vi "Vision Processing - Test.vi"(8 "error in (no error)":errorcluster, 11 "Image Size":T1=enum."320x240") -> ()   [LabVIEW 2016]
uses:
  Vision Support Code/Camera Types.ctl
  <vilib>/Rock Robotics/WPI/Camera/WPI_CameraImageSize.ctl
  <vilib>/Rock Robotics/WPI/Camera/WPI_CameraWhite Balance Values.ctl
  <vilib>/Rock Robotics/WPI/Camera/WPI_CameraExposure Values.ctl
  <vilib>/Rock Robotics/WPI/Camera/WPI_CameraFrameRate.ctl
  TestBuild/Robot Global Data - Test.vi
  <vilib>/Rock Robotics/Network Tables/NT Write Number.vi
  <vilib>/vision/NI_Vision_Development_Module.lvlib
panel:
  in  "Image Size 2":T1=enum."320x240"
  out "loop ms":u32=74
  out "Calibration error":errorcluster={"status"=TRUE, "code"=-1074396113, "source"=""}
  in  "Display Original":bool
  in  "Display Mask":bool=TRUE
  in  "Line Border":cluster{"Top":dbl, "Bottom":dbl}={"Top"=6.0, "Bottom"=1.0}
  in  "Use Calibration":bool=TRUE
  out "Instructions:":string="Use Source to load image files from a directory, or use a USB or IP camera connected to your laptop. Use Camera Settings 1 and 2 to achieve a dark image with bright and colorful stripes.\nLED Color can encoded as HSL or related color modes. Calibrate to the same color as the strips being reflected to the camera.\nClick and draw a line in Original Image to auto-calibrate the LED Color. You may want to widen and tweak Sat and Val by hand.\nThe Annotate button affects drawing a rectangle around the stripes and labeling it with a distance in ft. Distance relies on knowing the Camera Type and lens calibration (it looks up the lens view angle).\n\nAdjust Score Cutoff to make the code more or less picky. If the color is not very unique, you may need to increase the number of particles considered. The diagram uses a Size Limit to ignore colored things that are too small. You may need to adjust it if you are targetting from far away.\n\nResults give you the distance to the target, the center and box in a normalized (-1 to 1) and pixel coordinates.\n\nBe sure to read about setting camera exposure and brightness to help simplify your image and acquire color saturated images.\n\nThere are lots of comments on the diagram to explain the code."
  in  "Color Mode":u16(ring)=3 items=["RGB", "HSL", "HSV", "HSI"]
  in  "Particles":dbl=5.0
  in  "Score Cutoff %":dbl=70.0
  in  "Camera Type":T2=enum."MS HD3000 square"
  out "Results":T3={"Distance (ft)"=inf, "Score"=-inf, "Normalized"={"Center"={-0.565625, 0.37083333333333335}, "Rectangle"={"Numeric"=-inf, "Numeric 2"=inf, "Numeric 3"=-inf, "Numeric 5"=inf}}, "Pixels"={"Center"={69.5, 75.5}, "Rectangle"={"Numeric"=-inf, "Numeric 2"=-inf, "Numeric 3"=-inf, "Numeric 5"=-inf}}} {"Score" format="%#_3g"; "Pixels"."Rectangle"."Numeric 5" format="%#_3g"; "Pixels"."Rectangle"."Numeric 3" format="%#_3g"; "Pixels"."Rectangle"."Numeric 2" format="%#_3g"; "Pixels"."Rectangle"."Numeric" format="%#_3g"; "Normalized"."Rectangle"."Numeric 5" format="%#_2g"; "Normalized"."Rectangle"."Numeric 3" format="%#_2g"; "Normalized"."Rectangle"."Numeric 2" format="%#_2g"; "Normalized"."Rectangle"."Numeric" format="%#_2g"; "Normalized"."Center"."?" format="%#_3g"; "Normalized"."Center"."?" format="%#_3g"; "Distance (ft)" format="%#_3g"}
  out "Qualified Particles":i32=1
  in  "LED Color":T4={"Hue"={46.852959751357716, 116.77171286119035}, "Sat"={0.0, 255.0}, "Val"={15.178571428571438, 255.0}} {"Hue" scale=0.0..255.0 scale format="%#_3g"}
  out "Mask":T5(plugin-control)
  out "Original Image":T5(plugin-control)
  # "Legend:\n    Rectangle\n       Green - Good target, distance ft\n       Red - Bad target\n    Orange Text - Score in %"
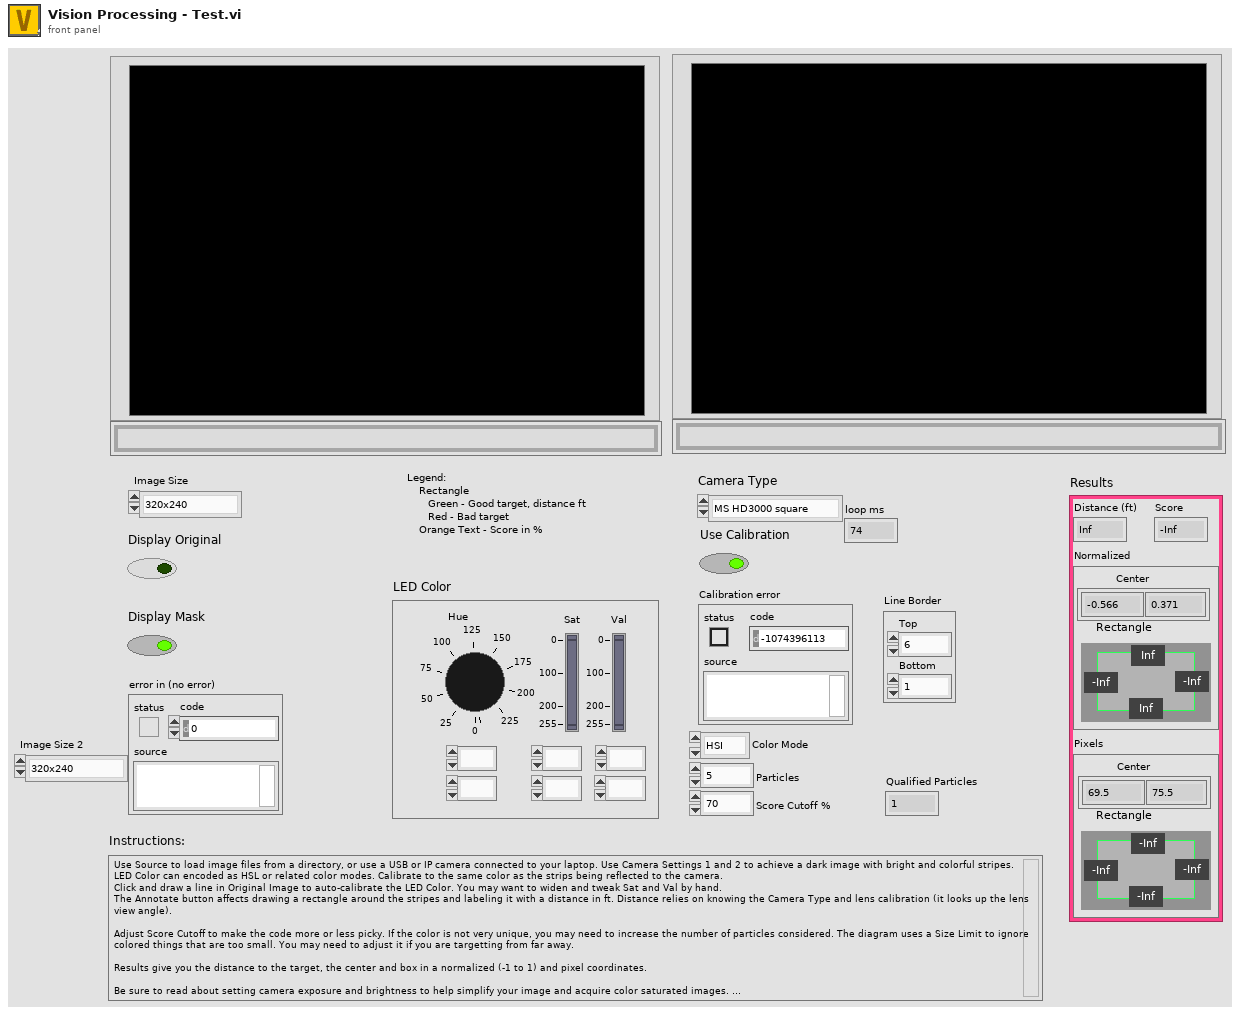
[diagram p1: front panel]
types:
  T1 = typedef "WPI_CameraImageSize.ctl" = enum16{"640x480", "320x240", "160x120", "Custom"}
  T2 = typedef "Camera Types.ctl" = enum16{"206", "1011", "1013", "MS HD3000 square", "MS HD3000 640x480"}
  T3 = cluster{"Distance (ft)":dbl, "Score":dbl, "Normalized":cluster{"Center":cluster{dbl, dbl}, "Rectangle":cluster{"Numeric":dbl, "Numeric 2":dbl, "Numeric 3":dbl, "Numeric 5":dbl}}, "Pixels":cluster{"Center":cluster{dbl, dbl}, "Rectangle":cluster{"Numeric":dbl, "Numeric 2":dbl, "Numeric 3":dbl, "Numeric 5":dbl}}}
  T4 = cluster{"Hue":cluster{dbl, dbl}, "Sat":cluster{dbl, dbl}, "Val":cluster{dbl, dbl}}
  T5 = typedef "IMAQ Image.ctl" = refnum<image>
  T6 = typedef "WPI_CameraFrameRate.ctl" = u32
  T7 = typedef "WPI_CameraExposure Values.ctl" = enum16{"Auto", "Flicker-free 50 Hz", "Flicker-free 60 Hz", "Hold current", "Custom"}
  T8 = typedef "WPI_CameraWhite Balance Values.ctl" = enum16{"Auto", "Fixed indoor", "Fixed outdoor 1", "Fixed outdoor 2", "Fixed fluorescent 1", "Fixed fluorescent 2", "Hold current", "Custom"}
  T9 = typedef "Image Type" = u32
  T10 = typedef "Particle Parameters" = i32
  T11 = typedef "WPI_CameraDevRef.ctl" = cluster{"Camera Address":string, "CameraStatus":errorcluster}
  T12 = cluster{"Left":dbl, "Top":dbl, "Right":dbl, "Bottom":dbl}
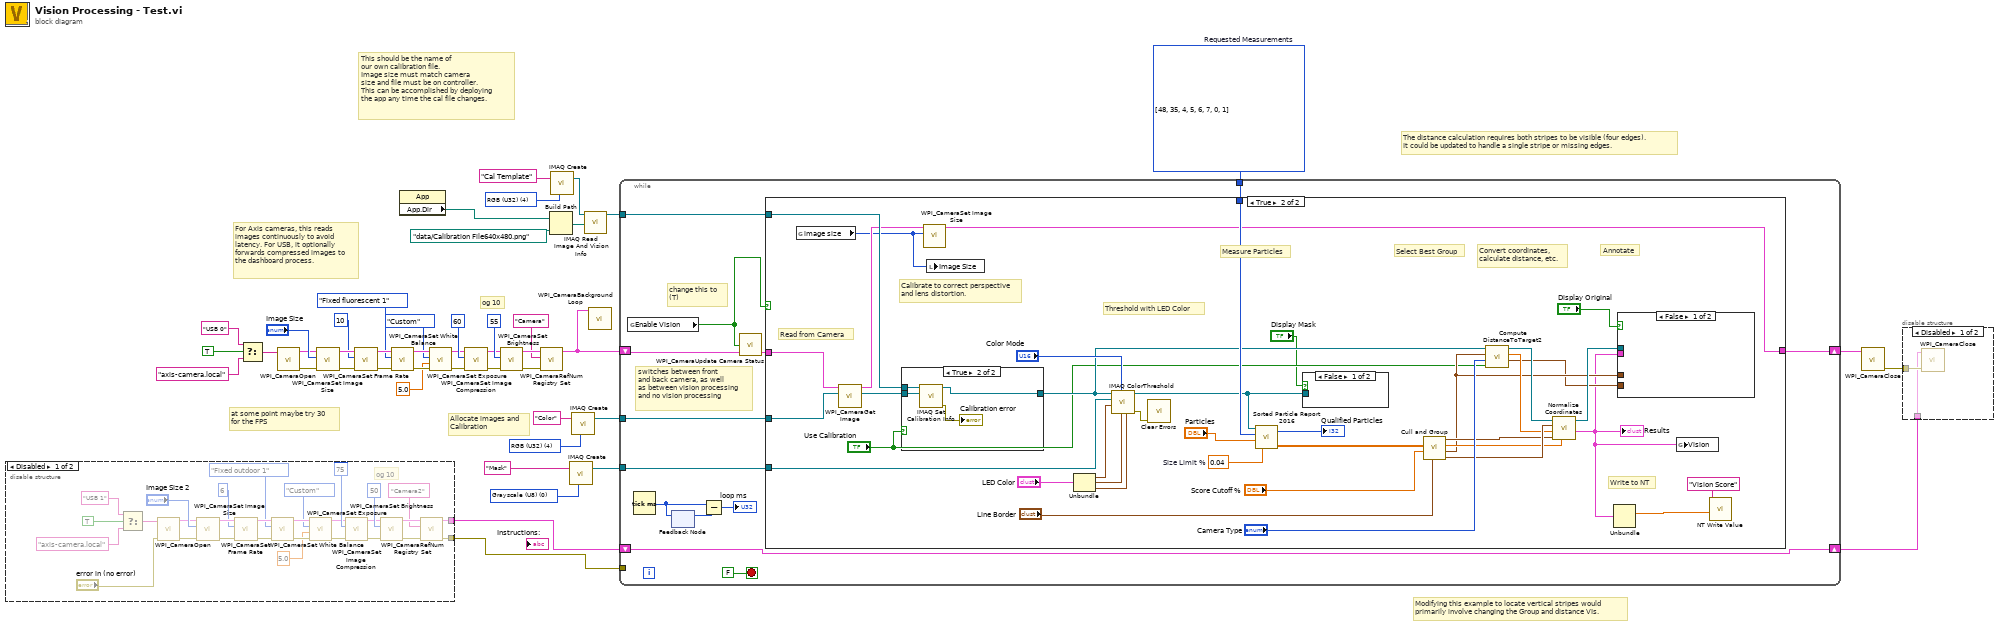
[diagram p0: block diagram]
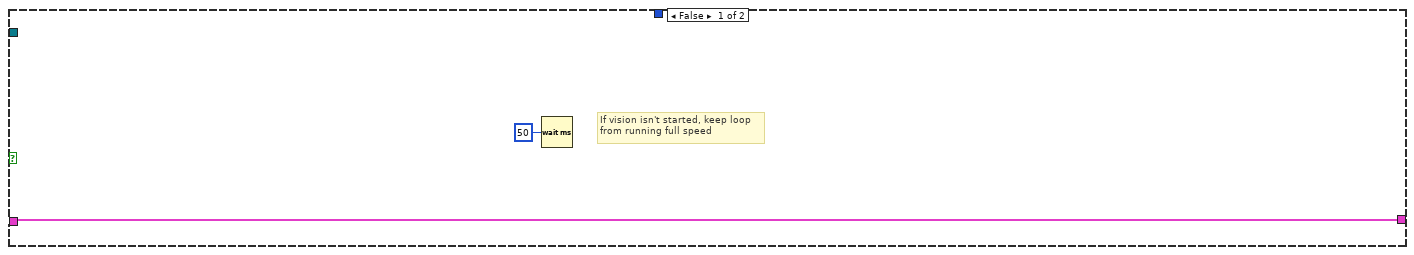
[diagram p4: hidden frame]
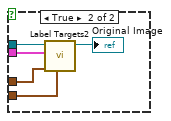
[diagram p5: hidden frame]
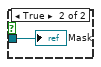
[diagram p6: hidden frame]
diagram:
  w39 = T9 4 items=["Grayscale (U8)", "Grayscale (I16)", "Grayscale (SGL)", "Complex (CSG)", "RGB (U32)", "HSL (U32)", "RGB (U64)", "Grayscale (U16)"] ("Image Type")
  w41 = T10[] [48, 35, 4, 5, 6, 7, 0, 1] items=["Center of Mass X", "Center of Mass Y", "First Pixel X", "First Pixel Y", "Bounding Rect Left", "Bounding Rect Top", "Bounding Rect Right", "Bounding Rect Bottom", "Max Feret Diameter Start X", "Max Feret Diameter Start Y", "Max Feret Diameter End X", "Max Feret Diameter End Y", "Max Horiz. Segment Length Left", "Max Horiz. Segment Length Right", "Max Horiz. Segment Length Row", "-", "Bounding Rect Width", "Bounding Rect Height", "Bounding Rect Diagonal", "Perimeter", "Convex Hull Perimeter", "Holes' Perimeter", "Max Feret Diameter", "Equivalent Ellipse Major Axis", "Equivalent Ellipse Minor Axis", "Equivalent Ellipse Minor Axis (Feret)", "Equivalent Rect Long Side", "Equivalent Rect Short Side", "Equivalent Rect Diagonal", "Equivalent Rect Short Side (Feret)", "Average Horiz. Segment Length", "Average Vert. Segment Length", "Hydraulic Radius", "Waddel Disk Diameter", "-", "Area", "Holes' Area", "Particle & Holes' Area", "Convex Hull Area", "Image Area", "-", "Number of Holes", "Number of Horiz. Segments", "Number of Vert. Segments", "-", "Orientation", "Max Feret Diameter Orientation", "-", "% Area/Image Area", "% Area/(Particle & Holes' Area)", "Ratio of Equivalent Ellipse Axes", "Ratio of Equivalent Rect Sides", "-", "Elongation Factor", "Compactness Factor", "Heywood Circularity Factor", "Type Factor", "-", "Sum X", "Sum Y", "Sum XX", "Sum XY", "Sum YY", "Sum XXX", "Sum XXY", "Sum XYY", "Sum YYY", "-", "Moment of Inertia XX", "Moment of Inertia XY", "Moment of Inertia YY", "Moment of Inertia XXX", "Moment of Inertia XXY", "Moment of Inertia XYY", "Moment of Inertia YYY", "Norm. Moment of Inertia XX", "Norm. Moment of Inertia XY", "Norm. Moment of Inertia YY", "Norm. Moment of Inertia XXX", "Norm. Moment of Inertia XXY", "Norm. Moment of Inertia XYY", "Norm. Moment of Inertia YYY", "Hu Moment 1", "Hu Moment 2", "Hu Moment 3", "Hu Moment 4", "Hu Moment 5", "Hu Moment 6", "Hu Moment 7"]  # Requested Measurements
  w44 = T9 0 items=["Grayscale (U8)", "Grayscale (I16)", "Grayscale (SGL)", "Complex (CSG)", "RGB (U32)", "HSL (U32)", "RGB (U64)", "Grayscale (U16)"] ("Image Type")
  w45 = T9 4 items=["Grayscale (U8)", "Grayscale (I16)", "Grayscale (SGL)", "Complex (CSG)", "RGB (U32)", "HSL (U32)", "RGB (U64)", "Grayscale (U16)"] ("Image Type")
  # "og 10"
  # "at some point maybe try 30 \nfor the FPS"
  # "This should be the name of \nour own calibration file.\nImage size must match camera\nsize and file must be on controller.\nThis can be accomplished by deploying\nthe app any time the cal file changes."
  # "For Axis cameras, this reads\nimages continuously to avoid\nlatency. For USB, it optionally\nforwards compressed images to\nthe dashboard process."
  # "Modifying this example to locate vertical stripes would\nprimarily involve changing the Group and distance VIs."
  # "The distance calculation requires both stripes to be visible (four edges).\nIt could be updated to handle a single stripe or missing edges."
  # "Allocate images and\nCalibration"
  n1 = disable-structure shown="Disabled" {
    disable-tunnel: [w49 _] -> w4
    disable-tunnel: [w47 _] -> w2
    frame Disabled {
      # "og 10"
      n2 = Select(t="USB 1" ("format string"), s=TRUE ("dot notation? (F)"), f="axis-camera.local" ("format string")) -> (s? t:f=w51:string)
      n3 = call <vilib>:"WPI_CameraOpen.vi"("error in (no error)"="error in (no error)", "Camera Address"=w51) -> ("error out"=w63:errorcluster, "CameraDevRef"=w64:T11)  [unwired: 8 out]
      n4 = call <vilib>:"WPI_CameraSet Image Size.vi"("error in (no error)"=w63, "Image Size"="Image Size 2", "CameraDevRef"=w64) -> ("error out"=w62:errorcluster, "CameraDevRef Out"=w65:T11)  [unwired: 1 in, 6 out]
      n5 = call <vilib>:"WPI_CameraSet Frame Rate.vi"("error in (no error)"=w62, "Frame Rate (fps)"=T6 6, "CameraDevRef"=w65) -> ("error out"=w61:errorcluster, "CameraDevRef Out"=w67:T11)  [unwired: 7 out]
      n6 = call <vilib>:"WPI_CameraSet White Balance.vi"("error in (no error)"=w61, "White Balance"=WPI_CameraWhite_Balance_Values."Fixed outdoor 1", "CameraDevRef"=w67) -> ("error out"=w60:errorcluster, "CameraDevRef Out"=w66:T11)  [unwired: 1 in, 6 out]
      n7 = call <vilib>:"WPI_CameraSet Exposure.vi"("error in (no error)"=w60, "Exposure (%)"=5.0, "Exposure"=WPI_CameraExposure_Values."Custom", "CameraDevRef"=w66) -> ("error out"=w59:errorcluster, "CameraDevRef Out"=w69:T11)  [unwired: 6 out]
      n8 = call <vilib>:"WPI_CameraSet Image Compression.vi"("error in (no error)"=w59, "Compression"=75, "CameraDevRef"=w69) -> ("error out"=w58:errorcluster, "CameraDevRef Out"=w68:T11)  [unwired: 7 out]
      n9 = call <vilib>:"WPI_CameraSet Brightness.vi"("error in (no error)"=w58, "Brightness"=50, "CameraDevRef"=w68) -> ("error out"=w57:errorcluster, "CameraDevRef Out"=w75:T11)  [unwired: 7 out]
      n10 = call <vilib>:"WPI_CameraRefNum Registry Set.vi"("error in (no error)"=w57, "refnum name"="Camera2", "CameraDevRef"=w75) -> ("error out"=w49:errorcluster, "CameraDevRef"=w47:T11)  [unwired: 1 in, 6 out]
    }
    frame Enabled {
    }
  }
  n11 = Select(t="USB 0" ("format string"), s=TRUE ("dot notation? (F)"), f="axis-camera.local" ("format string")) -> (s? t:f=w9:string)
  n12 = call <vilib>:"WPI_CameraOpen.vi"("Camera Address"=w9) -> ("error out"=w21:errorcluster, "CameraDevRef"=w22:T11)  [unwired: 1 in, 8 out]
  n13 = call <vilib>:"WPI_CameraSet Image Size.vi"("error in (no error)"=w21, "Image Size"="Image Size", "CameraDevRef"=w22) -> ("error out"=w20:errorcluster, "CameraDevRef Out"=w23:T11)  [unwired: 1 in, 6 out]
  n14 = call <vilib>:"WPI_CameraSet Frame Rate.vi"("error in (no error)"=w20, "Frame Rate (fps)"=T6 10, "CameraDevRef"=w23) -> ("error out"=w19:errorcluster, "CameraDevRef Out"=w25:T11)  [unwired: 7 out]
  n15 = call <vilib>:"WPI_CameraSet White Balance.vi"("error in (no error)"=w19, "White Balance"=WPI_CameraWhite_Balance_Values."Fixed fluorescent 1", "CameraDevRef"=w25) -> ("error out"=w18:errorcluster, "CameraDevRef Out"=w24:T11)  [unwired: 1 in, 6 out]
  n16 = property class="App"() -> ("App.Dir"=w5:path)  [unwired: 2 in, 2 out]
  n17 = call <vilib>:"WPI_CameraSet Exposure.vi"("error in (no error)"=w18, "Exposure (%)"=5.0, "Exposure"=WPI_CameraExposure_Values."Custom", "CameraDevRef"=w24) -> ("error out"=w17:errorcluster, "CameraDevRef Out"=w27:T11)  [unwired: 6 out]
  n18 = call <vilib>:"WPI_CameraSet Image Compression.vi"("error in (no error)"=w17, "Compression"=60, "CameraDevRef"=w27) -> ("error out"=w16:errorcluster, "CameraDevRef Out"=w26:T11)  [unwired: 7 out]
  n19 = call <vilib>:"WPI_CameraSet Brightness.vi"("error in (no error)"=w16, "Brightness"=55, "CameraDevRef"=w26) -> ("error out"=w15:errorcluster, "CameraDevRef Out"=w33:T11)  [unwired: 7 out]
  n20 = call <vilib>:"WPI_CameraRefNum Registry Set.vi"("error in (no error)"=w15, "refnum name"="Camera", "CameraDevRef"=w33) -> ("CameraDevRef"=w8:T11)  [unwired: 1 in, 7 out]
  n21 = Build Path(base path=w5, name or relative path=path "data/Calibration File640x480.png" ("Folder Location")) -> (appended path=w35:path)
  n22 = call "IMAQ Create"("Image Name"="Cal Template", "Image Type"=w39) -> ("New Image"=w37:T5)  [unwired: 2 in, 2 out]
  n23 = call "IMAQ Create"("Image Name"="Mask", "Image Type"=w44) -> ("New Image"=w42:T5)  [unwired: 2 in, 2 out]
  n24 = call "IMAQ Create"("Image Name"="Color", "Image Type"=w45) -> ("New Image"=w40:T5)  [unwired: 2 in, 2 out]
  n25 = call "IMAQ Read Image And Vision Info"("File Path"=w35, "Image"=w37) -> ("Image Out"=w36:T5)  [unwired: 7 in, 2 out]
  n26 = call <vilib>:"WPI_CameraBackground Loop.vi"("CameraDevRef"=w8) -> ()  [unwired: 11 in]
  n27 = while {
    tunnel: w40 -> [w84]
    tunnel: w42 -> [w87]
    tunnel: w41 -> [w86]
    tunnel: w36 -> [w85]
    shift-right: [w83] -> w7
    shift-left: w8 -> [w82]
    tunnel: w4 -> [_]
    shift-right: [w76] -> w1
    shift-left: w2 -> [w76]
    stop <- FALSE stop-if-true
    # "change this to \n(T)"
    # "switches between front\nand back camera, as well \nas between vision processing \nand no vision processing"
    n28 = global read "Robot Global Data - Test.vi" "Enable Vision"() -> (w77:bool)
    n29 = Tick Count (ms)() -> (millisecond timer value=w79:u32)
    n30 = feedback-in #1(w79) -> ()
    n31 = feedback #1() -> (w80:u32)  [unwired: 1 in]
    n32 = Subtract(x=w79, y=w80) -> (x-y=→"loop ms":u32)
    n33 = call <vilib>:"WPI_CameraUpdate Camera Status.vi"("CameraDevRef In"=w82, "Enable Vision"=w77) -> ("CameraDevRef Out"=w81:T11)  [unwired: 3 in]
    n34 = case shown="True" w77 {
      tunnel: w87 -> [_ w128]
      tunnel: w86 -> [_ w124]
      tunnel: w85 -> [_ w104]
      tunnel: w81 -> [w90 w101]
      tunnel: w84 -> [_ w100]
      tunnel: [w90 w95] -> w83
      frame False {
        # "If vision isn't started, keep loop\nfrom running full speed"
        n35 = Wait (ms)(milliseconds to wait=u32 50) -> ()  [unwired: 1 out]
      }
      frame True {
        w122 = 0.04  # Size Limit %
        # "Write to NT"
        # "Read from Camera"
        # "Calibrate to correct perspective\nand lens distortion."
        # "Measure Particles"
        # "Convert coordinates,\ncalculate distance, etc."
        # "Annotate"
        # "Select Best Group"
        # "Threshold with LED Color"
        n36 = global read "Robot Global Data - Test.vi" "image size"() -> (w94:T1)
        n37 = call <vilib>:"WPI_CameraGet Image.vi"("Image"=w100, "CameraDevRef"=w101) -> ("Image Out"=w99:T5, "CameraDevRef Out"=w96:T11)  [unwired: 7 in, 1 out]
        n38 = case shown="True" "Use Calibration" {
          tunnel: [w135 w139] -> w105
          tunnel: w99 -> [w135 w138]
          tunnel: w104 -> [_ w137]
          frame False {
          }
          frame True {
            n39 = call "IMAQ Set Calibration Info"("Image Dst"=w138, "Image Src"=w137) -> ("error out"=→"Calibration error":errorcluster, "Calibrated Image"=w139:T5)  [unwired: 8 in]
          }
        }
        n40 = call <vilib>:"WPI_CameraSet Image Size.vi"("Image Size"=w94, "CameraDevRef"=w96) -> ("CameraDevRef Out"=w95:T11)  [unwired: 2 in, 7 out]
        n41 = local write "Image Size"(w94) -> ()
        n42 = Unbundle("LED Color") -> ("Hue"=w127:cluster{dbl, dbl}, "Sat"=w126:cluster{dbl, dbl}, "Val"=w125:cluster{dbl, dbl})
        n43 = call "IMAQ ColorThreshold"("Blue or Luma or Val or Inten Range"=w125, "Green or Sat Range"=w126, "Color Mode"="Color Mode", "Red or Hue Range"=w127, "Image Dst"=w128, "Image Src"=w105) -> ("error out"=w121:errorcluster, "Image Dst Out"=w117:T5)  [unwired: 4 in]
        n44 = call <vilib>:"Clear Errors.vi"("error in (no error)"=w121) -> ()  [unwired: 5 in, 2 out]
        n45 = call "Sorted Particle Report 2016.vi"("Min Area Size %"=w122, "Particle Count Limit"="Particles", "Pixel Measurements"=w124, "Image in"=w117) -> ("Sorted Data"=w119:dbl[][], "Particles"=→"Qualified Particles":i32)
        n46 = case shown="False" "Display Mask" {
          tunnel: w117 -> [_ w134]
          frame False {
          }
          frame True {
            "Mask" <- w134
          }
        }
        n47 = call "Cull and Group.vi"("Line Border"="Line Border", "Score Cutoff"="Score Cutoff %", "Sorted Data"=w119) -> ("Rect"=w115:T12, "Line"=w107:T12, "Score"=w110:dbl, "Center"=w111:cluster{"X":dbl, "Y":dbl})  [unwired: 5 in]
        n48 = call "Compute DistanceToTarget2.vi"("Calibrated"="Use Calibration", "Camera Type"="Camera Type", "Line"=w107, "Image Src"=w105) -> ("Edges"=w106:cluster{"X":sgl, "Y":sgl}[], "Distance (ft)"=w114:dbl, "Image Dst Out"=w113:T5)  [unwired: 5 in]
        n49 = call "Normalize Coordinates.vi"("Score"=w110, "Center"=w111, "Distance"=w114, "Bounding box"=w115, "Image in"=w113) -> ("Results"=w91:T3, "Image out"=w112:T5)  [unwired: 5 in]
        "Results" <- w91
        n50 = Unbundle(w91) -> ("Score"=w93:dbl)  [unwired: 3 out]
        n51 = case shown="False" "Display Original" {
          tunnel: w112 -> [_ w132]
          tunnel: w91 -> [_ w131]
          tunnel: w107 -> [_ w130]
          tunnel: w106 -> [_ w129]
          frame False {
          }
          frame True {
            n52 = call "Label Targets2.vi"("Edges"=w129, "Line"=w130, "Results"=w131, "Image in"=w132) -> ("Image out"=→"Original Image":T5)  [unwired: 7 in]
          }
        }
        n53 = global write "Robot Global Data - Test.vi" "Vision"(w91) -> ()
        n54 = call-poly <vilib>:"NT Write Value.vi"("Numeric"=w93, "Name"="Vision Score") -> ()  [unwired: 9 in, 1 out]
      }
    }
  }
  n55 = call <vilib>:"WPI_CameraClose.vi"("CameraDevRef"=w7) -> ("error out"=w3:errorcluster)  [unwired: 1 in, 9 out]
  n56 = disable-structure shown="Disabled" {
    disable-tunnel: w3 -> [w141 _]
    disable-tunnel: w1 -> [w140 _]
    frame Disabled {
      n57 = call <vilib>:"WPI_CameraClose.vi"("error in (no error)"=w141, "CameraDevRef"=w140) -> ()  [unwired: 10 out]
    }
    frame Enabled {
    }
  }
